vi "Remove the Items Under Compact Array.vi"(10 "ODs in":T1[](array[typedef]) {"SubNumber" format="%x"; "AccessType" items=["", "ro", "wo", "rw", "const", "rwr", "rww"]; "DataType" items=[""=0, "BOOLEAN"=1, "INTEGER8"=2, "INTEGER16"=3, "INTEGER32"=4, "UNSIGNED8"=5, "UNSIGNED16"=6, "UNSIGNED32"=7, "REAL32"=8, "VISIBLE_STRING"=9, "OCTET_STRING"=10, "UNICODE_STRING"=11, "TIME_OF_DAY"=12, "TIME_DIFFERENCE"=13, "DOMAIN"=15, "INTEGER24"=16, "REAL64"=17, "INTEGER40"=18, "INTEGER48"=19, "INTEGER56"=20, "INTEGER64"=21, "UNSIGNED24"=22, "UNSIGNED40"=24, "UNSIGNED48"=25, "UNSIGNED56"=26, "UNSIGNED64"=27]; "ObjectType" items=[""=10, "NULL"=0, "DOMAIN"=2, "DEFTYPE"=5, "DEFSTRUCT"=6, "VAR"=7, "ARRAY"=8, "RECORD"=9]; "sub-index" format="%x"; "index" format="%x"}, 11 "Index":i32) -> (2 "ODs out":T1[](array[typedef]) {"SubNumber" format="%x"; "AccessType" items=["", "ro", "wo", "rw", "const", "rwr", "rww"]; "DataType" items=[""=0, "BOOLEAN"=1, "INTEGER8"=2, "INTEGER16"=3, "INTEGER32"=4, "UNSIGNED8"=5, "UNSIGNED16"=6, "UNSIGNED32"=7, "REAL32"=8, "VISIBLE_STRING"=9, "OCTET_STRING"=10, "UNICODE_STRING"=11, "TIME_OF_DAY"=12, "TIME_DIFFERENCE"=13, "DOMAIN"=15, "INTEGER24"=16, "REAL64"=17, "INTEGER40"=18, "INTEGER48"=19, "INTEGER56"=20, "INTEGER64"=21, "UNSIGNED24"=22, "UNSIGNED40"=24, "UNSIGNED48"=25, "UNSIGNED56"=26, "UNSIGNED64"=27]; "ObjectType" items=[""=10, "NULL"=0, "DOMAIN"=2, "DEFTYPE"=5, "DEFSTRUCT"=6, "VAR"=7, "ARRAY"=8, "RECORD"=9]; "sub-index" format="%x"; "index" format="%x"}, 3 "Next Index":i32)   [LabVIEW 2013]
uses:
  control/OD Entry.ctl
  control/Object Type.ctl
  control/Data Type.ctl
  control/Access Type.ctl
  control/OD Cateory.ctl
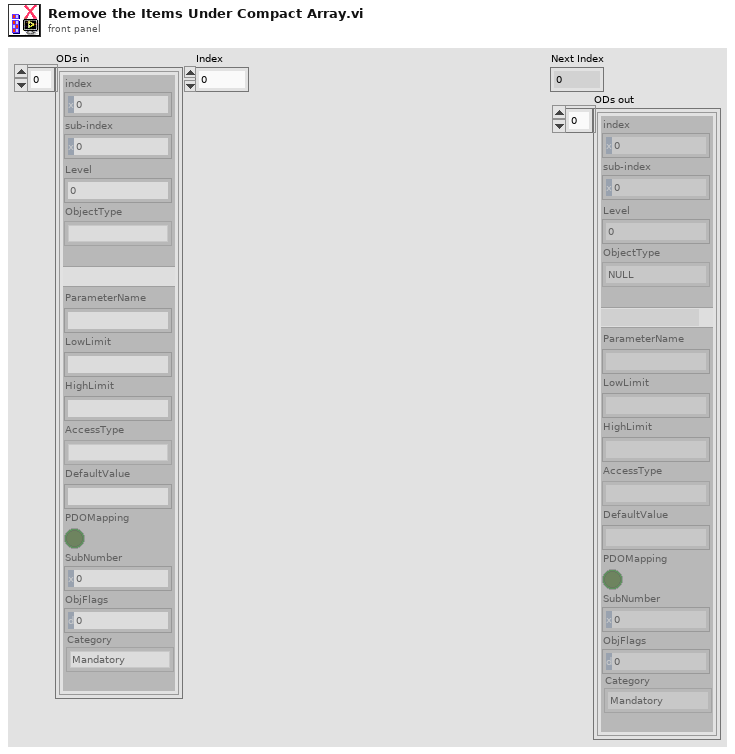
[diagram p1: front panel]
types:
  T1 = typedef "OD Entry.ctl" = cluster{"index":u16, "sub-index":u8, "Level":u8, "ObjectType":T2, "DataType":T3, "ParameterName":string, "LowLimit":string, "HighLimit":string, "AccessType":T4, "DefaultValue":string, "PDOMapping":bool, "SubNumber":u8, "ObjFlags":u32, "Category":T5}
  T2 = typedef "Object Type.ctl" = u16
  T3 = typedef "Data Type.ctl" = u16
  T4 = typedef "Access Type.ctl" = u16
  T5 = typedef "OD Cateory.ctl" = enum16{"Mandatory", "Optional", "Manufacturer", ""}
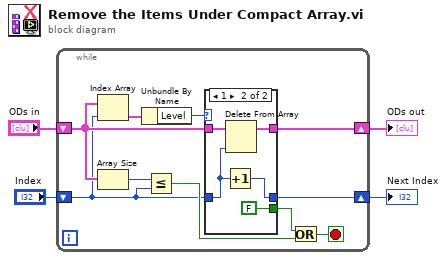
[diagram p0: block diagram]
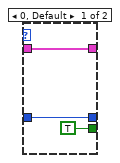
[diagram p2: hidden frame]
diagram:
  n1 = while {
    shift-right: [w5] -> w2
    shift-left: "Index" -> [w6]
    shift-right: [w8] -> w1
    shift-left: "ODs in" -> [w9]
    stop <- w13 stop-if-true
    n2 = Index Array(array=w9, index=w6) -> (element=w11:T1)
    n3 = Array Size(array=w9) -> (size(s)=w14:i32)
    n4 = Unbundle By Name(w11) -> ("Level"=w10:u8)
    n5 = Less Or Equal?(x=w14, y=w6) -> (x <= y?=w12:bool)
    n6 = case shown="1" w10 {
      tunnel: w9 -> [w17 w22]
      tunnel: [w17 w21] -> w8
      tunnel: w6 -> [w15 w19]
      tunnel: [TRUE FALSE] -> w7
      tunnel: [w15 w18] -> w5
      frame 0, Default {
      }
      frame 1 {
        n7 = Increment(x=w19) -> (x+1=w18:i32)
        n8 = Delete From Array(array=w22, index=w19) -> (array with subset deleted=w21:T1[])  [unwired: 1 in, 1 out]
      }
    }
    n9 = Or(x=w7, y=w12) -> (x .or. y?=w13:bool)
  }
  "Next Index" <- w2
  "ODs out" <- w1
